vi "niRFUtil RFHS Channelizer DesignFFTResampler.vi"(0 "Channel fs":dbl, 2 "Benchmark Task":T1, 11 "error in (no error)":errorcluster, 12 "fft2Size":i32=2048) -> (4 "fft1Descriptors":u64[](array[numeric]), 6 "fft2Descriptors":u64[](array[numeric]), 8 "Buffer Size":i32, 14 "fft1Size":i32, 15 "error out":errorcluster)   [LabVIEW 2015, in "niRFUtil.lvlib"]
uses:
  niRFUtil.lvlib
  Utilities/Benchmark/niRFUtil RFHS Benchmark Task.ctl
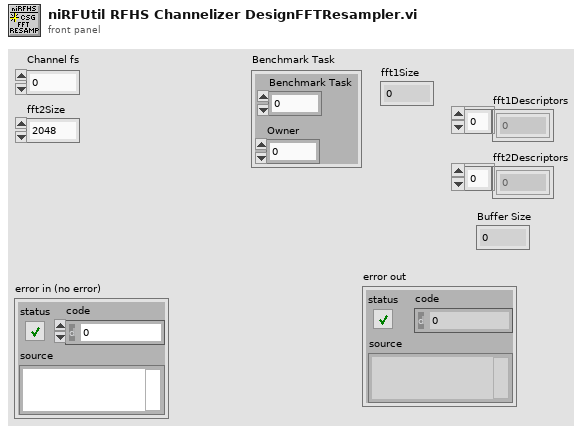
[diagram p1: front panel]
types:
  T1 = typedef "niRFUtil.lvlib/niRFUtil RFHS Benchmark Task.ctl" = cluster{"Benchmark Task":u64, "Owner":u32}
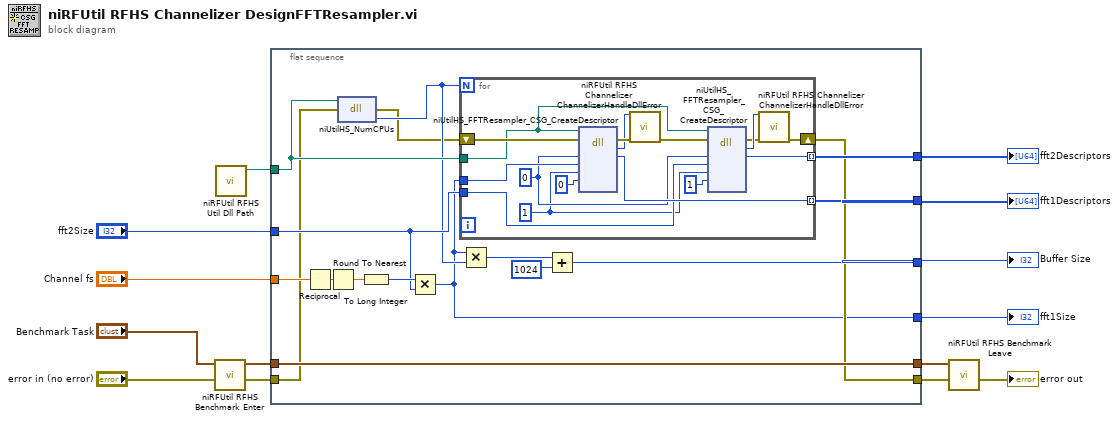
[diagram p0: block diagram]
diagram:
  n1 = call "niRFUtil RFHS Benchmark Enter.vi"("error in (no error)"="error in (no error)", "Benchmark Task (Parent)"="Benchmark Task") -> ("error out"=w5:errorcluster, "Benchmark Task (Self)"=w10:T1)  [unwired: 8 in]
  n2 = call "niRFUtil RFHS Util Dll Path.vi"() -> ("Path"=w7:path)  [unwired: 7 in, 4 out]
  n3 = flat-sequence {
    tunnel: "Channel fs" -> [w21]
    tunnel: [w31] -> w13
    tunnel: [w30] -> w2
    tunnel: "fft2Size" -> [w24]
    tunnel: w10 -> [w23]
    tunnel: [w23] -> w9
    tunnel: [w22] -> w8
    tunnel: w7 -> [w19]
    tunnel: w5 -> [w17]
    tunnel: [w20] -> w3
    tunnel: [w15] -> w1
    frame #0 {
      n4 = Reciprocal(x=w21) -> (1/x=w25:dbl)
      n5 = Round To Nearest(number=w25) -> (nearest integer value=w27:dbl)
      n6 = dll-call lib="?" fn="niUtilHS_NumCPUs"(path in=w19, error in=w17) -> (error out=w16:errorcluster, "return type"=w18:i32)  [unwired: 1 in, 1 out]
      n7 = To Long Integer(number=w27) -> (32bit integer=w26:i32)
      n8 = Multiply(x=w26, y=w24) -> (x*y=w15:i32)
      n9 = for {
        N: w18 -> [_]
        tunnel: [w47] -> w31 mode=indexing
        tunnel: w15 -> [w46]
        tunnel: [w45] -> w30 mode=indexing
        tunnel: w24 -> [w44]
        shift-right: [w32] -> w20
        shift-left: w16 -> [w39]
        tunnel: w19 -> [w38]
        w40 = u32 1 ("inverse")
        w42 = u64 0 ("dsc")
        n10 = dll-call lib="?" fn="niUtilHS_FFTResampler_CSG_CreateDescriptor"(path in=w38, error in=w39, "dsc"=w42, "fftSize"=w46, "shift"=w40, "inverse"=u32 0) -> (error out=w37:errorcluster, "return type"=w36:i32, "dsc"=w47:u64)  [unwired: 6 in, 1 out]
        n11 = call "niRFUtil RFHS Channelizer ChannelizerHandleDllError.vi"("Error"=w36, "error in (no error)"=w37) -> ("error out"=w35:errorcluster)  [unwired: 13 in]
        n12 = dll-call lib="?" fn="niUtilHS_FFTResampler_CSG_CreateDescriptor"(path in=w38, error in=w35, "dsc"=w42, "fftSize"=w44, "shift"=w40, "inverse"=u32 1 ("shift")) -> (error out=w33:errorcluster, "return type"=w34:i32, "dsc"=w45:u64)  [unwired: 6 in, 1 out]
        n13 = call "niRFUtil RFHS Channelizer ChannelizerHandleDllError.vi"("Error"=w34, "error in (no error)"=w33) -> ("error out"=w32:errorcluster)  [unwired: 13 in]
      }
      n14 = Multiply(x=w15, y=w18) -> (x*y=w29:i32)
      n15 = Add(x=w29, y=1024) -> (x+y=w22:i32)
    }
  }
  n16 = call "niRFUtil RFHS Benchmark Leave.vi"("error in (no error)"=w3, "Benchmark Task Self"=w9) -> ("error out"=→"error out":errorcluster)  [unwired: 8 in, 1 out]
  "fft1Descriptors" <- w13
  "fft2Descriptors" <- w2
  "Buffer Size" <- w8
  "fft1Size" <- w1
